vi "Error Query.vi"(8 "error in (no error)":errorcluster, 11 "VISA resource name":refnum<visa-resource-name>) -> (0 "error out":errorcluster, 3 "VISA resource name out":refnum<visa-resource-name>, 4 "Device Errors":cluster{"code":i32, "Text":string}[](array[cluster]))   [LabVIEW 2014, in "Stanford Research DG645 - Driver.lvlib"]
doc: "Status and Display Command: LERR?\n\nQueries the instrument for any errors in the instrument's error queue. It will continue to read errors until all errors have been read from the instrument. Any errors will be returned in the error out control.\n\n<B>Note:</B>\nThis VI is called automatically by all driver VIs so it is not necessary to call this in an application."
uses:
  Stanford Research DG645 - Driver.lvlib
panel:
  in  "Device Error":cluster{"code":i32, "Text":string}
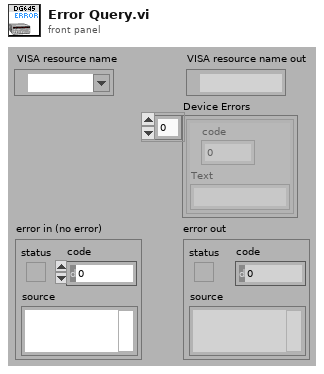
[diagram p1: front panel]
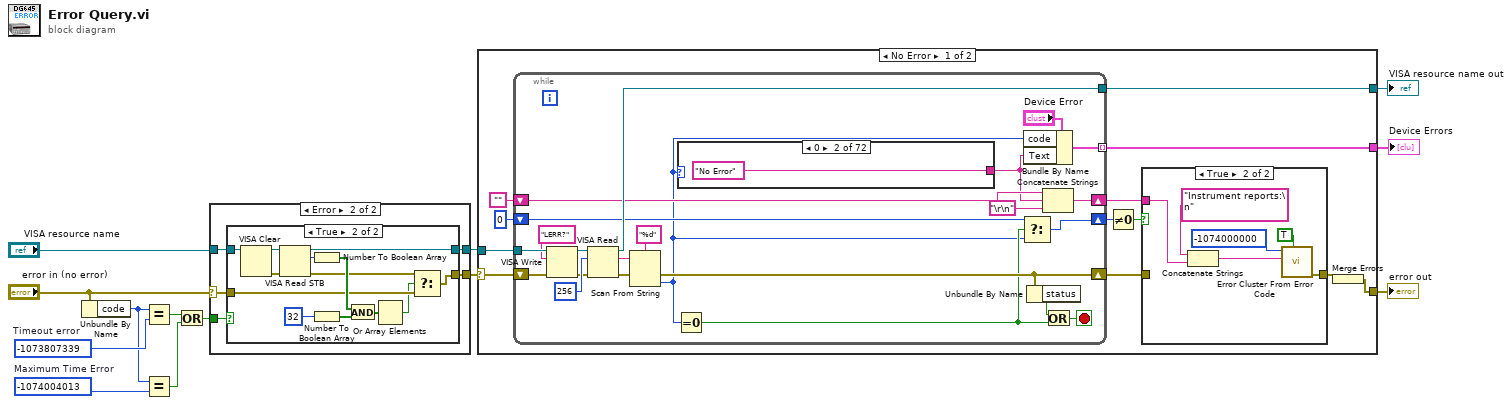
[diagram p0: block diagram]
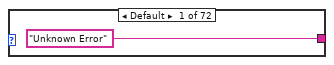
[diagram p5: hidden frame]
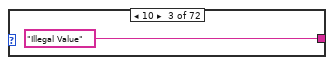
[diagram p6: hidden frame]
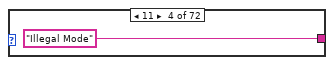
[diagram p7: hidden frame]
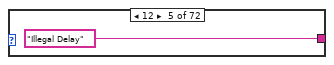
[diagram p8: hidden frame]
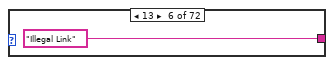
[diagram p9: hidden frame]
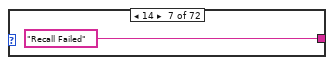
[diagram p10: hidden frame]
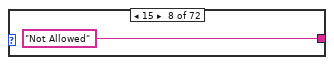
[diagram p11: hidden frame]
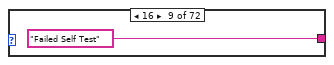
[diagram p12: hidden frame]
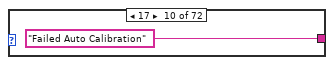
[diagram p13: hidden frame]
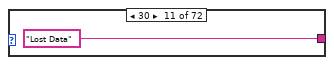
[diagram p14: hidden frame]
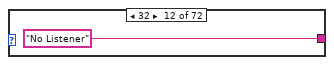
[diagram p15: hidden frame]
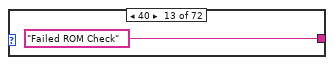
[diagram p16: hidden frame]
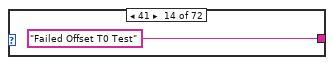
[diagram p17: hidden frame]
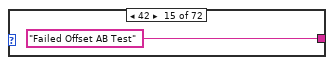
[diagram p18: hidden frame]
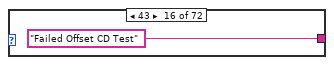
[diagram p19: hidden frame]
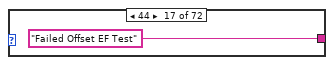
[diagram p20: hidden frame]
diagram:
  w6 = -1074004013  # Maximum Time Error
  w8 = -1073807339  # Timeout error
  n1 = Unbundle By Name("error in (no error)") -> ("code"=w7:i32)
  n2 = Equal?(x=w7, y=w8) -> (x = y?=w4:bool)
  n3 = Equal?(x=w7, y=w6) -> (x = y?=w5:bool)
  n4 = Or(x=w4, y=w5) -> (x .or. y?=w3:bool)
  n5 = case shown="Error" "error in (no error)" {
    selector: "error in (no error)" -> [w14 w18]
    tunnel: "VISA resource name" -> [w15 w20]
    tunnel: [w15 w19] -> w10
    tunnel: [w14 w17] -> w11
    tunnel: w3 -> [_ w16]
    frame No Error {
    }
    frame Error {
      n6 = case shown="True" w16 {
        tunnel: w20 -> [w22 w28]
        tunnel: [w22 w25] -> w19
        tunnel: w18 -> [w21 w31]
        tunnel: [w21 w30] -> w17
        frame False {
        }
        frame True {
          n7 = VISA Clear(VISA resource name=w28) -> (VISA resource name out=w27:refnum<visa-resource-name>, error out=w26:errorcluster)  [unwired: 1 in]
          n8 = VISA Read STB(8:w26, 11:w27) -> (0:w24:errorcluster, 2:w23:u16, 3:w25:refnum<visa-resource-name>)
          n9 = Number To Boolean Array(number=w23) -> (Boolean array=w32:bool[])
          n10 = Number To Boolean Array(number=32) -> (Boolean array=w34:bool[])
          n11 = And(x=w32, y=w34) -> (x .and. y?=w33:bool[])
          n12 = Or Array Elements(Boolean array=w33) -> (logical OR=w29:bool)
          n13 = Select(t=w24, s=w29, f=w31) -> (s? t:f=w30:errorcluster)
        }
      }
    }
  }
  n14 = case shown="No Error" w11 {
    selector: w11 -> [w36 w151]
    tunnel: [w47 w152] -> w13
    tunnel: w10 -> [w46 w152]
    tunnel: [w44 w151] -> w12
    tunnel: [w38 cluster{"code":i32, "Text":string}[] []] -> w1
    frame No Error {
      n15 = while {
        tunnel: [w77] -> w47
        tunnel: w46 -> [w76]
        shift-right: [w67] -> w39
        shift-left: "" -> [w69]
        shift-right: [w65] -> w40
        shift-left: 0 -> [w66]
        shift-right: [w63] -> w37
        shift-left: w36 -> [w64]
        tunnel: [w57] -> w38 mode=indexing
        stop <- w70 stop-if-true
        n16 = VISA Write(VISA resource name=w76, write buffer="LERR?" ("Error Query Command"), error in (no error)=w64) -> (VISA resource name out=w75:refnum<visa-resource-name>, error out=w73:errorcluster)  [unwired: 1 out]
        n17 = VISA Read(VISA resource name=w75, byte count=u32 256 ("Bytes"), error in (no error)=w73) -> (VISA resource name out=w77:refnum<visa-resource-name>, read buffer=w60:string, error out=w61:errorcluster)  [unwired: 1 out]
        n18 = Scan From String(format string="%d", input string=w60, error in=w61) -> (error out=w63:errorcluster, output 1=w56:i32)  [unwired: 2 in, 2 out]
        n19 = Equal To 0?(x=w56) -> (x = 0?=w59:bool)
        n20 = case shown="0" w56 {
          tunnel: ["Unknown Error" "No Error" "Illegal Value" "Illegal Mode" "Illegal Delay" "Illegal Link" "Recall Failed" "Not Allowed" "Failed Self Test" "Failed Auto Calibration" "Lost Data" "No Listener" "Failed ROM Check" "Failed Offset T0 Test" "Failed Offset AB Test" "Failed Offset CD Test" "Failed Offset EF Test" "Failed Offset GH Test" "Failed Amplitude T0 Test" "Failed Amplitude AB Test" "Failed Amplitude CD Test" "Failed Amplitude EF Test" "Failed Amplitude GH Test" "Failed FPGA Communications Test" "Failed GPIB Communications Test" "Failed DDS Communications Test" "Failed Serial EEPROM Communications Test" "Failed Temperature Sensor Communications Test" "Failed PLL Communications Test" "Failed DAC 0 Communications Test" "Failed DAC 1 Communications Test" "Failed DAC 2 Communications Test" "Failed Sample and Hold Operations Test" "Failed Vjitter Operations Test" "Failed Channel T0 Analog Delay Test" "Failed Channel T1 Analog Delay Test" "Failed Channel A Analog Delay Test" "Failed Channel B Analog Delay Test" "Failed Channel C Analog Delay Test" "Failed Channel D Analog Delay Test" "Failed Channel E Analog Delay Test" "Failed Channel F Analog Delay Test" "Failed Channel G Analog Delay Test" "Failed Channel H Analog Delay Test" "Failed Sample and Hold Calibration" "Failed T0 Calibration" "Failed T1 Calibration" "Failed A Calibration" "Failed B Calibration" "Failed C Calibration" "Failed D Calibration" "Failed E Calibration" "Failed F Calibration" "Failed G Calibration" "Failed H Calibration" "Failed Vjitter Calibration" "Illegal Command" "Undefined Command" "Illegal Query" "Illegal Set" "Null Parameter" "Extra Parameters" "Missing Parameters" "Parameter Overflow" "Invalid Floating Point Number" "Invalid Integer" "Integer Overflow" "Invalid Hexadecimal" "Syntax Error" "Communication Error" "Over Run" "Too Many Errors"] -> w55
          frame Default {
          }
          frame 0 {
          }
          frame 10 {
          }
          frame 11 {
          }
          frame 12 {
          }
          frame 13 {
          }
          frame 14 {
          }
          frame 15 {
          }
          frame 16 {
          }
          frame 17 {
          }
          frame 30 {
          }
          frame 32 {
          }
          frame 40 {
          }
          frame 41 {
          }
          frame 42 {
          }
          frame 43 {
          }
          frame 44 {
          }
          frame 45 {
          }
          frame 46 {
          }
          frame 47 {
          }
          frame 48 {
          }
          frame 49 {
          }
          frame 50 {
          }
          frame 51 {
          }
          frame 52 {
          }
          frame 53 {
          }
          frame 54 {
          }
          frame 55 {
          }
          frame 56 {
          }
          frame 57 {
          }
          frame 58 {
          }
          frame 59 {
          }
          frame 60 {
          }
          frame 61 {
          }
          frame 62 {
          }
          frame 63 {
          }
          frame 64 {
          }
          frame 65 {
          }
          frame 66 {
          }
          frame 67 {
          }
          frame 68 {
          }
          frame 69 {
          }
          frame 70 {
          }
          frame 71 {
          }
          frame 80 {
          }
          frame 81 {
          }
          frame 82 {
          }
          frame 83 {
          }
          frame 84 {
          }
          frame 85 {
          }
          frame 86 {
          }
          frame 87 {
          }
          frame 88 {
          }
          frame 89 {
          }
          frame 90 {
          }
          frame 91 {
          }
          frame 110 {
          }
          frame 111 {
          }
          frame 112 {
          }
          frame 113 {
          }
          frame 114 {
          }
          frame 115 {
          }
          frame 116 {
          }
          frame 117 {
          }
          frame 118 {
          }
          frame 120 {
          }
          frame 121 {
          }
          frame 122 {
          }
          frame 126 {
          }
          frame 170 {
          }
          frame 171 {
          }
          frame 254 {
          }
        }
        n21 = Select(t=w66, s=w59, f=w56) -> (s? t:f=w65:i32)
        n22 = Bundle By Name(cluster="Device Error", "code"=w56, "Text"=w55) -> (w57:cluster{"code":i32, "Text":string})
        n23 = Unbundle By Name(w63) -> ("status"=w62:bool)
        n24 = Concatenate Strings(w69, w55, "\r\n") -> (w67:string)
        n25 = Or(x=w62, y=w59) -> (x .or. y?=w70:bool)
      }
      n26 = Not Equal To 0?(x=w40) -> (x != 0?=w42:bool)
      n27 = case shown="True" w42 {
        tunnel: w39 -> [_ w53]
        tunnel: [w48 w49] -> w41
        tunnel: w37 -> [w48 _]
        frame False {
        }
        frame True {
          n28 = Concatenate Strings("Instrument reports:\n" ("Source"), w53) -> (w50:string)
          n29 = call <vilib>:"Error Cluster From Error Code.vi"("show call chain? (False)"=TRUE, "error message (\"\")"=w50, "error code (0)"=-1074000000 ("Code")) -> ("error out"=w49:errorcluster)  [unwired: 6 in]
        }
      }
      n30 = Merge Errors(w41) -> (w44:errorcluster)
    }
    frame Error {
      (unwired) i32[] []
      (unwired) ""
    }
  }
  "VISA resource name out" <- w13
  "error out" <- w12
  "Device Errors" <- w1
